vi "Pneumatic Test.vi"(11 "ProgressText":string) -> (2 "EndTestText":string)   [LabVIEW 2012]
uses:
  <vilib>/Rock Robotics/WPI/Compressor/WPI_CompressorGetSetRefNum.vi
panel:
  in  "Timeout (ms)":i32=60000
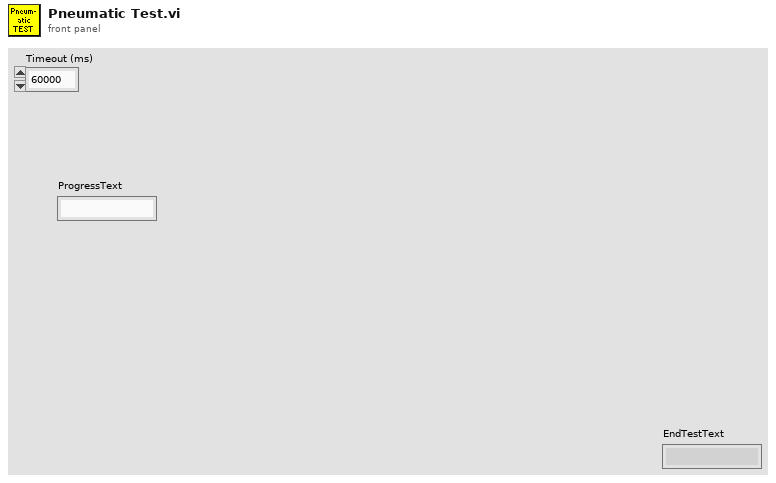
[diagram p1: front panel]
types:
  T1 = typedef "WPI_CompressorDevRef.ctl" = cluster{"DevStatus":errorcluster, "DigitalInputDevRef":T2, "RelayDevRef":T5}
  T2 = typedef "WPI_DigitalInputDevRef.ctl" = cluster{"DevStatus":errorcluster, "DIO Channel":T3, "Digital Module":T4}
  T3 = typedef "FPGA_DIOChannel.ctl" = enum8{"DIO 1", "DIO 2", "DIO 3", "DIO 4", "DIO 5", "DIO 6", "DIO 7", "DIO 8", "DIO 9", "DIO 10", "DIO 11", "DIO 12", "DIO 13", "DIO 14", "Invalid"}
  T4 = typedef "FPGA_TypedefDigitalModule.ctl" = enum16{"Digital Module 1", "Digital Module 2"}
  T5 = typedef "WPI_RelayDevRef.ctl" = cluster{"DevStatus":errorcluster, "Relay Channel":T6, "Digital Module":T4, "Relay Direction":T7}
  T6 = typedef "FPGA_DIORelayChannel.ctl" = enum8{"Relay 1", "Relay 2", "Relay 3", "Relay 4", "Relay 5", "Relay 6", "Relay 7", "Relay 8", "Invalid"}
  T7 = typedef "WPI_RelayDirection.ctl" = enum16{"Both directions", "Forward only", "Reverse only"}
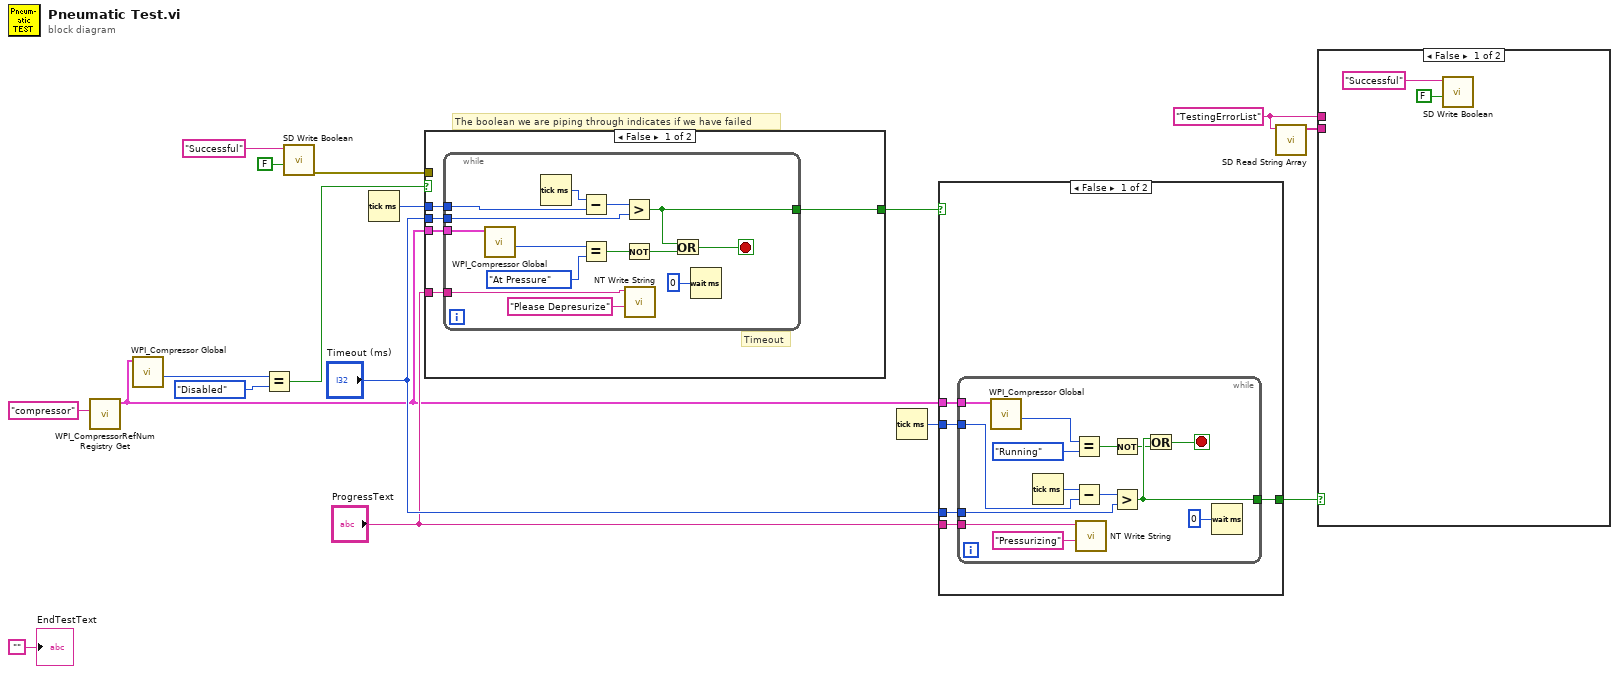
[diagram p0: block diagram]
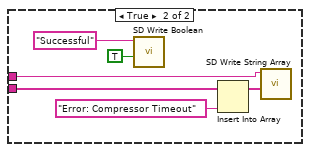
[diagram p2: hidden frame]
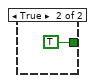
[diagram p4: hidden frame]
diagram:
  w4 = "TestingErrorList" ("Name")
  # "The boolean we are piping through indicates if we have failed"
  n1 = call <vilib>:"WPI_CompressorRefNum Registry Get.vi"("refnum name"="compressor") -> ("CompressorDevRef"=w7:T1)  [unwired: 9 in, 1 out]
  n2 = call <vilib>:"WPI_Compressor Global.vi"("CompressorDevRef"=w7) -> ("Compressor State Out"=w16:enum16{"Disabled", "Running", "At Pressure"})  [unwired: 9 in, 1 out]
  n3 = Equal?(x=w16, y=enum16{"Disabled", "Running", "At Pressure"}."Disabled") -> (x = y?=w12:bool)
  n4 = call <vilib>:"SD Write Boolean.vi"("Boolean"=FALSE, "Name"="Successful") -> ("error out"=w1:errorcluster)  [unwired: 8 in, 1 out]
  n5 = Tick Count (ms)() -> (millisecond timer value=w14:u32)
  n6 = case shown="False" w12 {
    tunnel: w14 -> [w22 _]
    tunnel: "Timeout (ms)" -> [w21 _]
    tunnel: "ProgressText" -> [w20 _]
    tunnel: w7 -> [w19 _]
    tunnel: [w18 TRUE] -> w11
    tunnel: w1 -> [_ _]
    frame False {
      # "Timeout"
      n7 = while {
        tunnel: w22 -> [w35]
        tunnel: w21 -> [w33]
        tunnel: w20 -> [w31]
        tunnel: [w25] -> w18
        tunnel: w19 -> [w29]
        stop <- w23 stop-if-true
        n8 = call <vilib>:"WPI_Compressor Global.vi"("CompressorDevRef"=w29) -> ("Compressor State Out"=w28:enum16{"Disabled", "Running", "At Pressure"})  [unwired: 9 in, 1 out]
        n9 = Tick Count (ms)() -> (millisecond timer value=w36:u32)
        n10 = Subtract(x=w36, y=w35) -> (x-y=w34:u32)
        n11 = Equal?(x=w28, y=enum16{"Disabled", "Running", "At Pressure"}."At Pressure" ("Compressor State Out")) -> (x = y?=w26:bool)
        n12 = Greater?(x=w34, y=w33) -> (0:w25:bool)
        n13 = Not(x=w26) -> (.not. x?=w24:bool)
        n14 = call <vilib>:"NT Write String.vi"("String"="Please Depresurize", "Name"=w31) -> ()  [unwired: 9 in, 1 out]
        n15 = Or(x=w25, y=w24) -> (x .or. y?=w23:bool)
        n16 = Wait (ms)(milliseconds to wait=u32 0) -> ()  [unwired: 1 out]
      }
    }
    frame True {
    }
  }
  n17 = Tick Count (ms)() -> (millisecond timer value=w10:u32)
  n18 = case shown="False" w11 {
    selector: w11 -> [_ w57]
    tunnel: [w38 w57] -> w6
    tunnel: w10 -> [w42 _]
    tunnel: "Timeout (ms)" -> [w41 _]
    tunnel: "ProgressText" -> [w40 _]
    tunnel: w7 -> [w39 _]
    frame False {
      n19 = while {
        tunnel: w42 -> [w55]
        tunnel: w41 -> [w53]
        tunnel: w40 -> [w51]
        tunnel: [w45] -> w38
        tunnel: w39 -> [w49]
        stop <- w43 stop-if-true
        n20 = call <vilib>:"WPI_Compressor Global.vi"("CompressorDevRef"=w49) -> ("Compressor State Out"=w48:enum16{"Disabled", "Running", "At Pressure"})  [unwired: 9 in, 1 out]
        n21 = Tick Count (ms)() -> (millisecond timer value=w56:u32)
        n22 = Equal?(x=w48, y=enum16{"Disabled", "Running", "At Pressure"}."Running" ("Compressor State Out")) -> (x = y?=w46:bool)
        n23 = Subtract(x=w56, y=w55) -> (x-y=w54:u32)
        n24 = call <vilib>:"NT Write String.vi"("String"="Pressurizing", "Name"=w51) -> ()  [unwired: 9 in, 1 out]
        n25 = Not(x=w46) -> (.not. x?=w44:bool)
        n26 = Greater?(x=w54, y=w53) -> (0:w45:bool)
        n27 = Or(x=w45, y=w44) -> (x .or. y?=w43:bool)
        n28 = Wait (ms)(milliseconds to wait=u32 0) -> ()  [unwired: 1 out]
      }
    }
    frame True {
    }
  }
  n29 = call <vilib>:"SD Read String Array.vi"("Name"=w4) -> ("String Array"=w5:string[])  [unwired: 9 in, 1 out]
  n30 = case shown="False" w6 {
    tunnel: w5 -> [_ w65]
    tunnel: w4 -> [_ w63]
    frame False {
      n31 = call <vilib>:"SD Write Boolean.vi"("Boolean"=FALSE, "Name"="Successful") -> ()  [unwired: 8 in, 2 out]
    }
    frame True {
      n32 = call <vilib>:"SD Write Boolean.vi"("Boolean"=TRUE, "Name"="Successful") -> ()  [unwired: 8 in, 2 out]
      n33 = Insert Into Array(array=w65, new element="Error: Compressor Timeout" ("new element/subarray")) -> (w62:string[])  [unwired: 1 in]
      n34 = call <vilib>:"SD Write String Array.vi"("String Array"=w62, "Name"=w63) -> ()  [unwired: 8 in, 2 out]
    }
  }
  "EndTestText" <- ""
